vi "PSDLorentianFit_NODECIMATION_array_input.vi"(7 "High frequency cutoff %":dbl=50.0, 9 "resample interval":dbl=1.3, 10 "dt [s]":dbl=0.0001, 11 "signal":dbl[](array[numeric])) -> (0 "best fit parameters from resampled data":dbl[](array[numeric])=[0.0019817222678975522, 691.5237834685465], 1 "k domain resampled":cluster{dbl[], "best nonlinear fit":dbl[]}[](graph), 2 "frequency domain info":T1, 3 "Time domain info":T2)   [LabVIEW 2020, in "CylinderCalibration.lvlib"]
uses:
  CylinderCalibration.lvlib
  <vilib>/Analysis/2dsp.llb/Real FFT.vi
  <vilib>/Analysis/baseanly.llb/Mean (DBL).vi
  <vilib>/gmath/NumericalOptimization/Nonlinear Curve Fit LM formula string.vi
  <vilib>/Analysis/NI_AALBase.lvlib
  <vilib>/Analysis/NI_AALPro.lvlib
  <vilib>/gmath/NI_Gmath.lvlib
panel:
  # "Fitting options:"
  # "0.000227068"
  # "0.000238785"
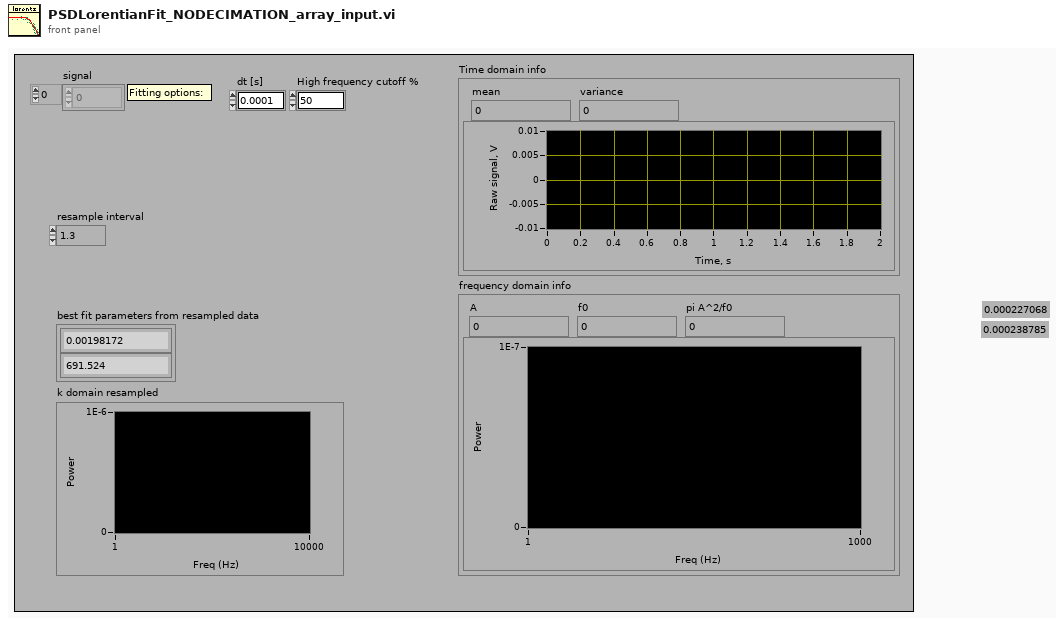
[diagram p1: front panel]
types:
  T1 = cluster{"A":dbl, "f0":dbl, "pi A^2/f0":dbl, "k domain":cluster{dbl[], "best nonlinear fit":dbl[]}[]}
  T2 = cluster{"mean":dbl, "variance":dbl, cluster{dbl[], "all rows":dbl[]}}
  T3 = cluster{"model":string, "Parameters":string[], "x":string}
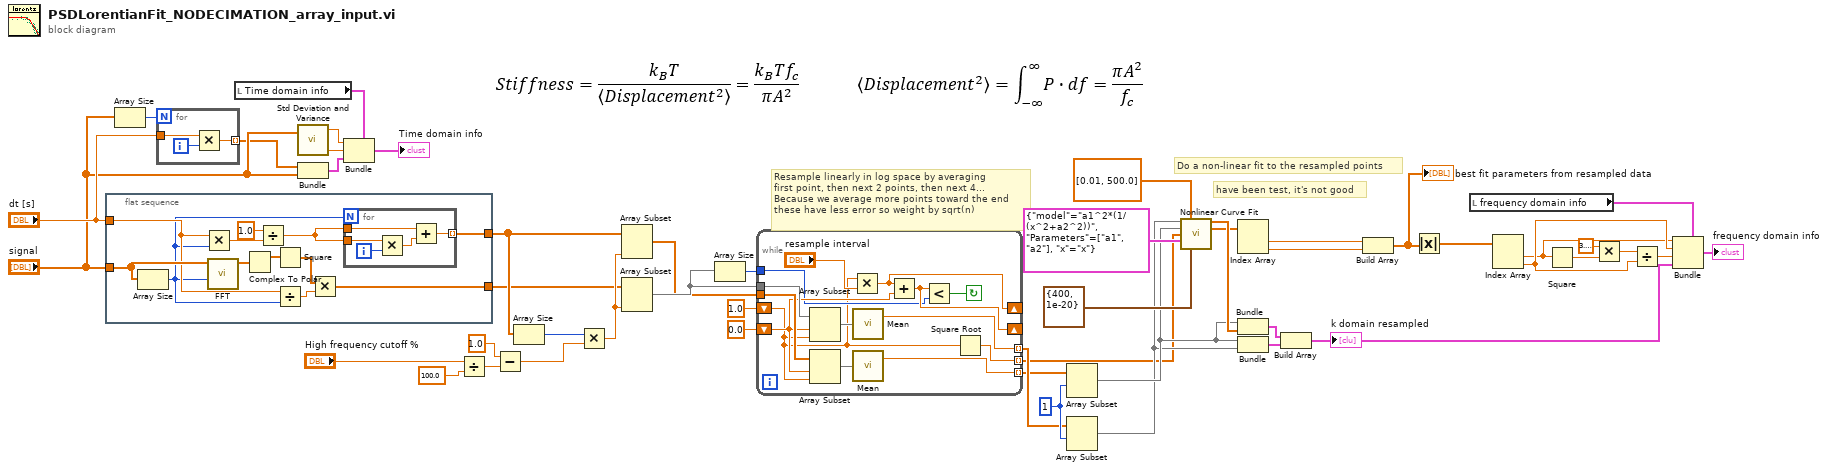
[diagram p0: block diagram]
diagram:
  w36 = 1 ("index")
  # "have been test, it's not good"
  # "Do a non-linear fit to the resampled points"
  # "Resample linearly in log space by averaging\nfirst point, then next 2 points, then next 4... \nBecause we average more points toward the end\nthese have less error so weight by sqrt(n)"
  n1 = flat-sequence {
    tunnel: "dt [s]" -> [w54]
    tunnel: "signal" -> [w59]
    tunnel: [w56] -> w6
    tunnel: [w50] -> w7
    frame #0 {
      n2 = Array Size(array=w59) -> (size(s)=w52:i32)
      n3 = Multiply(x=w54, y=w52) -> (x*y=w60:dbl)
      n4 = call-poly <vilib>:"FFT.vi"("FFT size"=w52, "X"=w59) -> ("FFT {X}"=w55:cdb[])  [unwired: 8 in, 1 out]
      n5 = Complex To Polar(r * e^(i*theta)=w55) -> (r=w58:dbl[])  [unwired: 1 out]
      n6 = Divide(x=1.0 ("y"), y=w60) -> (x/y=w51:dbl)
      n7 = Square(x=w58) -> (x^2=w57:dbl[])
      n8 = Divide(x=w54, y=w52) -> (x/y=w53:dbl)
      n9 = Multiply(x=w57, y=w53) -> (x*y=w56:dbl[])
      n10 = for {
        N: w52 -> [_]
        tunnel: w51 -> [w63]
        tunnel: w51 -> [w65]
        tunnel: [w62] -> w50 mode=indexing
        i -> [w66]
        n11 = Multiply(x=w65, y=w66) -> (x*y=w64:dbl)
        n12 = Add(x=w63, y=w64) -> (x+y=w62:dbl)
      }
    }
  }
  n13 = Array Size(array="signal") -> (size(s)=w46:i32)
  n14 = for {
    N: w46 -> [_]
    tunnel: "dt [s]" -> [w68]
    tunnel: [w67] -> w33 mode=indexing
    i -> [w69]
    n15 = Multiply(x=w68, y=w69) -> (x*y=w67:dbl)
  }
  n16 = local read "Time domain info"() -> (w43:T2)
  n17 = call <vilib>:"Std Deviation and Variance.vi"("X"="signal") -> ("mean"=w37:dbl, "variance"=w39:dbl)  [unwired: 1 in, 1 out]
  n18 = Bundle(w33, "signal"="signal") -> (w45:cluster{dbl[], "signal":dbl[]})  [unwired: 1 in]
  n19 = Bundle(cluster=w43, "mean"=w37, "variance"=w39, w45) -> (→"Time domain info":T2)
  n20 = Divide(x="High frequency cutoff %", y=100.0) -> (x/y=w40:dbl)
  n21 = Subtract(x=1.0, y=w40) -> (x-y=w42:dbl)
  n22 = Array Size(array=w7) -> (size(s)=w35:i32)
  n23 = Multiply(x=w35, y=w42) -> (x*y=w34:dbl)
  n24 = Array Subset(array=w7, length=w34) -> (w8:dbl[])  [unwired: 1 in]
  n25 = Array Subset(array=w6, length=w34) -> (w9:dbl[])  [unwired: 1 in]
  n26 = Array Size(array=w9) -> (size(s)=w28:i32)
  n27 = while {
    shift-right: [w82] -> _
    shift-left: 1.0 -> [w71]
    shift-right: [w73] -> _
    shift-left: 0.0 -> [w79]
    tunnel: w8 -> [w81]
    tunnel: w9 -> [w80]
    tunnel: [w76] -> w4 mode=indexing
    tunnel: [w75] -> w5 mode=indexing
    tunnel: w28 -> [w72]
    tunnel: [w70] -> w1 mode=indexing
    stop <- w74 continue-if-true
    n28 = Array Subset(array=w80, index=w79, length=w71) -> (w78:dbl[])
    n29 = Array Subset(array=w81, index=w79, length=w71) -> (w77:dbl[])
    n30 = Multiply(x=w71, y="resample interval") -> (x*y=w82:dbl)
    n31 = call-poly <vilib>:"Mean.vi"("X"=w78) -> ("mean"=w75:dbl)  [unwired: 1 out]
    n32 = call-poly <vilib>:"Mean.vi"("X"=w77) -> ("mean"=w76:dbl)  [unwired: 1 out]
    n33 = Add(x=w82, y=w79) -> (x+y=w73:dbl)
    n34 = Less?(x=w73, y=w72) -> (x < y?=w74:bool)
    n35 = Square Root(x=w71) -> (sqrt(x)=w70:dbl)
  }
  n36 = Array Subset(array=w4, index=w36) -> (w3:dbl[])  [unwired: 1 in]
  n37 = Array Subset(array=w5, index=w36) -> (w2:dbl[])  [unwired: 1 in]
  n38 = call-poly <vilib>:"Nonlinear Curve Fit.vi"("Y"=w2, "initial parameters"=dbl[] [0.01, 500.0], "X"=w3, "Weight"=w1, "model description"=T3 {"model"="a1^2*(1/(x^2+a2^2))", "Parameters"=["a1", "a2"], "x"="x"}, "termination"=cluster{"max iteration":i32, "tolerance":dbl} {"max iteration"=400, "tolerance"=1e-20}) -> ("best nonlinear fit"=w31:dbl[], "best fit parameters"=w23:dbl[])  [unwired: 5 in, 3 out]
  n39 = Index Array(array=w23) -> (element #1=w13:dbl, element #2=w12:dbl)  [unwired: 2 in]
  n40 = Bundle(w3, "best nonlinear fit"=w31) -> (w24:cluster{dbl[], "best nonlinear fit":dbl[]})  [unwired: 1 in]
  n41 = Bundle(w3, w2) -> (w25:cluster{dbl[], dbl[]})  [unwired: 1 in]
  n42 = Build Array(w24, w25) -> (w10:cluster{dbl[], "best nonlinear fit":dbl[]}[])
  "k domain resampled" <- w10
  n43 = Build Array(w13, w12) -> (w11:dbl[])
  "best fit parameters from resampled data" <- w11
  n44 = Absolute Value(x=w11) -> (abs(x)=w14:dbl[])
  n45 = local read "frequency domain info"() -> (w19:T1)
  n46 = Index Array(array=w14) -> (element #1=w16:dbl, element #2=w18:dbl)  [unwired: 2 in]
  n47 = Square(x=w16) -> (x^2=w21:dbl)
  n48 = Multiply(x=3.141592653589793, y=w21) -> (x*y=w20:dbl)
  n49 = Divide(x=w20, y=w18) -> (x/y=w22:dbl)
  n50 = Bundle(cluster=w19, "A"=w16, "f0"=w18, "pi A^2/f0"=w22, "k domain"=w10) -> (→"frequency domain info":T1)
